vi "Assign Joint Ramping v2 Test.vi"(5 "Ramp Time [sec]":dbl=3.0, 6 "Vac Digital Cmd":i8, 7 "Robot In":i32, 8 "error in":errorcluster, 9 "Destination Posit Array [mm]":dbl[](array[numeric])=[0.0, 0.0, -3.0, 0.0], 11 "FPGA VI Reference In":refnum<k20>) -> (0 "error out":errorcluster, 3 "FPGA VI Reference Out":refnum<k20>)   [LabVIEW 2016]
uses:
  <vilib>/Analysis/1siggen.llb/Ramp Pattern by Samples.vi
  Subsystems/Global Variables.vi
  <vilib>/Analysis/NI_AALBase.lvlib
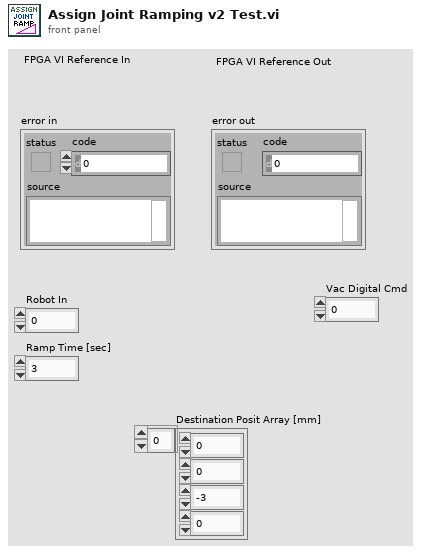
[diagram p1: front panel]
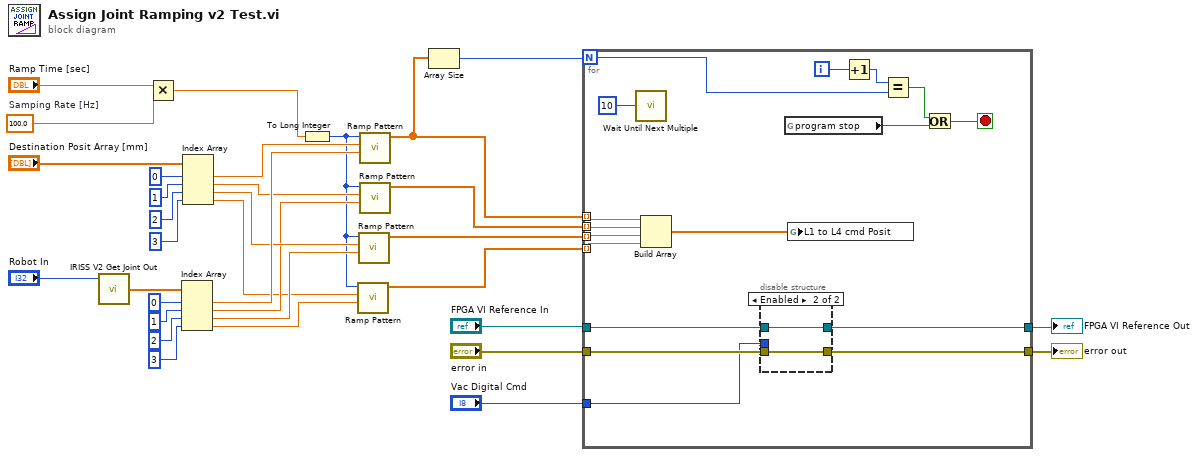
[diagram p0: block diagram]
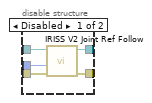
[diagram p2: hidden frame]
diagram:
  w23 = 100.0  # Samping Rate [Hz]
  n1 = call "IRISS V2 Get Joint Out.vi"("Left or Right Arm"="Robot In") -> ("Joint Out Posit"=w6:dbl[])  [unwired: 3 in, 1 out]
  n2 = Multiply(x="Ramp Time [sec]", y=w23) -> (x*y=w14:dbl)
  n3 = Index Array(array=w6, index #1=0 ("index"), index #2=1 ("index"), index #3=2 ("index"), index #4=3 ("index")) -> (element #1=w22:dbl, element #2=w18:dbl, element #3=w17:dbl, element #4=w16:dbl)
  n4 = Index Array(array="Destination Posit Array [mm]", index #1=0 ("index"), index #2=1 ("index"), index #3=2 ("index"), index #4=3 ("index")) -> (element #1=w21:dbl, element #2=w20:dbl, element #3=w19:dbl, element #4=w15:dbl)
  n5 = To Long Integer(number=w14) -> (32bit integer=w4:i32)
  n6 = call-poly <vilib>:"Ramp Pattern.vi"("start"=w16, "end"=w15, "samples"=w4) -> ("Ramp Pattern"=w11:dbl[])  [unwired: 7 in, 1 out]
  n7 = call-poly <vilib>:"Ramp Pattern.vi"("start"=w17, "end"=w19, "samples"=w4) -> ("Ramp Pattern"=w12:dbl[])  [unwired: 7 in, 1 out]
  n8 = call-poly <vilib>:"Ramp Pattern.vi"("start"=w22, "end"=w21, "samples"=w4) -> ("Ramp Pattern"=w3:dbl[])  [unwired: 7 in, 1 out]
  n9 = call-poly <vilib>:"Ramp Pattern.vi"("start"=w18, "end"=w20, "samples"=w4) -> ("Ramp Pattern"=w13:dbl[])  [unwired: 7 in, 1 out]
  n10 = Array Size(array=w3) -> (size(s)=w2:i32)
  n11 = for {
    N: w2 -> [w36]
    tunnel: w3 -> [w50] mode=indexing
    tunnel: w13 -> [w49] mode=indexing
    tunnel: w12 -> [w48] mode=indexing
    tunnel: w11 -> [w47] mode=indexing
    tunnel: "Vac Digital Cmd" -> [w34]
    tunnel: "FPGA VI Reference In" -> [w43]
    tunnel: [w44] -> w8
    tunnel: "error in" -> [w45]
    tunnel: [w46] -> w10
    i -> [w38]
    stop <- w40 stop-if-true
    n12 = call "Wait Until Next Multiple"("Count(mSec)"=u32 10) -> ()  [unwired: 1 out]
    n13 = Build Array(w50, w49, w48, w47) -> (w39:dbl[])
    n14 = disable-structure shown="Enabled" {
      disable-tunnel: [w55 w56] -> w46
      disable-tunnel: w45 -> [w54 w56]
      disable-tunnel: [w53 w57] -> w44
      disable-tunnel: w43 -> [w52 w57]
      disable-tunnel: w34 -> [w51 _]
      frame Disabled {
        n15 = call "IRISS V2 Joint Ref Follow.vi"("error in"=w54, "Digital Cmd [0-78]"=w51, "FPGA VI Reference In"=w52) -> ("error out"=w55:errorcluster, "FPGA VI Reference Out"=w53:refnum<k20>)  [unwired: 5 in]
      }
      frame Enabled {
      }
    }
    n16 = global read "Global Variables.vi" "program stop"() -> (w41:bool)
    n17 = global write "Global Variables.vi" "L1 to L4 cmd Posit"(w39) -> ()
    n18 = Increment(x=w38) -> (x+1=w37:i32)
    n19 = Equal?(x=w37, y=w36) -> (x = y?=w35:bool)
    n20 = Or(x=w35, y=w41) -> (x .or. y?=w40:bool)
  }
  "error out" <- w10
  "FPGA VI Reference Out" <- w8
